vi "Process Data XYGraph.vi"(5 "Queue":refnum<queue>) -> ()   [LabVIEW 2013, in "main.lvlib"]
uses:
  main.lvlib
  Controls/Enum Variables.ctl
  Controls/Enum User Events.ctl
  Controls/Enum Process Data.ctl
  CreatePDF XYGraph.vi
panel:
  out "Blue":cluster{"Pressure":dbl[], "Graph":dbl[]}(graph)
  out "Blue index":dbl format="%d%%"
  in  "ResetBlueBtn":bool
  in  "ZoomBlueBtn":bool
  out "Blue Pressure":dbl
  out "Red":cluster{"Pressure":dbl[], "Graph":dbl[]}(graph)
  out "Armpressure":dbl
  in  "System Stop Button":bool
  in  "GraphSelection(Red:F)":bool
  in  "Cursor Mode":bool
  in  "ResetFrontImage":bool
  out "Red index":dbl format="%d%%"
  out "Red Pressure":dbl
  in  "ResetRedBtn":bool
  in  "ZoomRedBtn":bool
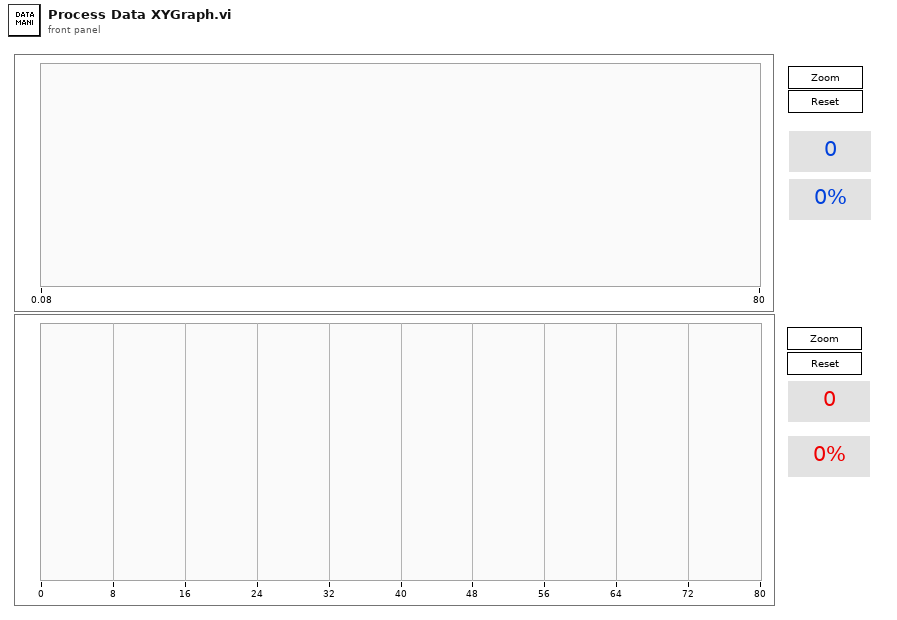
[diagram p1: front panel]
types:
  T1 = typedef "main.lvlib/Enum Process Data.ctl" = enum16{"Init", "Set Cursor Mode", "Set Data Path", "Get All"}
  T2 = typedef "main.lvlib/Enum Variables.ctl" = enum16{"SetAcqFilter", "GetAcqFilter", "Set Filter", "Get Filter", "Set Height", "Get Height", "Set Blue Pressure", "Get Blue Pressure", "Set Red Pressure", "Get Red Pressure", "Init", "Reset Pressure", "Set Red Cursors", "Get Red Cursors", "Set Blue Cursors", "Get Blue Cursors", "Set Language", "Get Language", "Set Active Graphs", "Get ActiveGraphs", "Set Method", "Get Method", "Set Encryption", "Get Encryption", "Set ExcelVersion", "Get ExcelVersion", "Set DICOM Avail", "Get DICOM Avail", "Set DICOM Encode", "Get DICOM Encode", "Set JournalExport", "Get JournalExport", "Set Sequence", "Get Sequence", "Set DAQ Connected", "Get DAQ Connected", "Set Current Graph", "Get Current Graph", "Set General Settings", "Get Hyphenation", "Set Arm Calc Method", "Get Arm Calc Method", "Set Dicom Tags", "Get Dicom Tags", "Set BT Serial", "Get BT Serial", "Set BT Accepted Serials", "Get BT Accepted Serials", "Get BT License", "Set BT License"}
  T3 = typedef "main.lvlib/Enum User Events.ctl" = enum16{"User Event", "Init"}
  T4 = typedef "LVPoint32TypeDef.ctl" = cluster{"Horizontal":i32, "Vertical":i32}
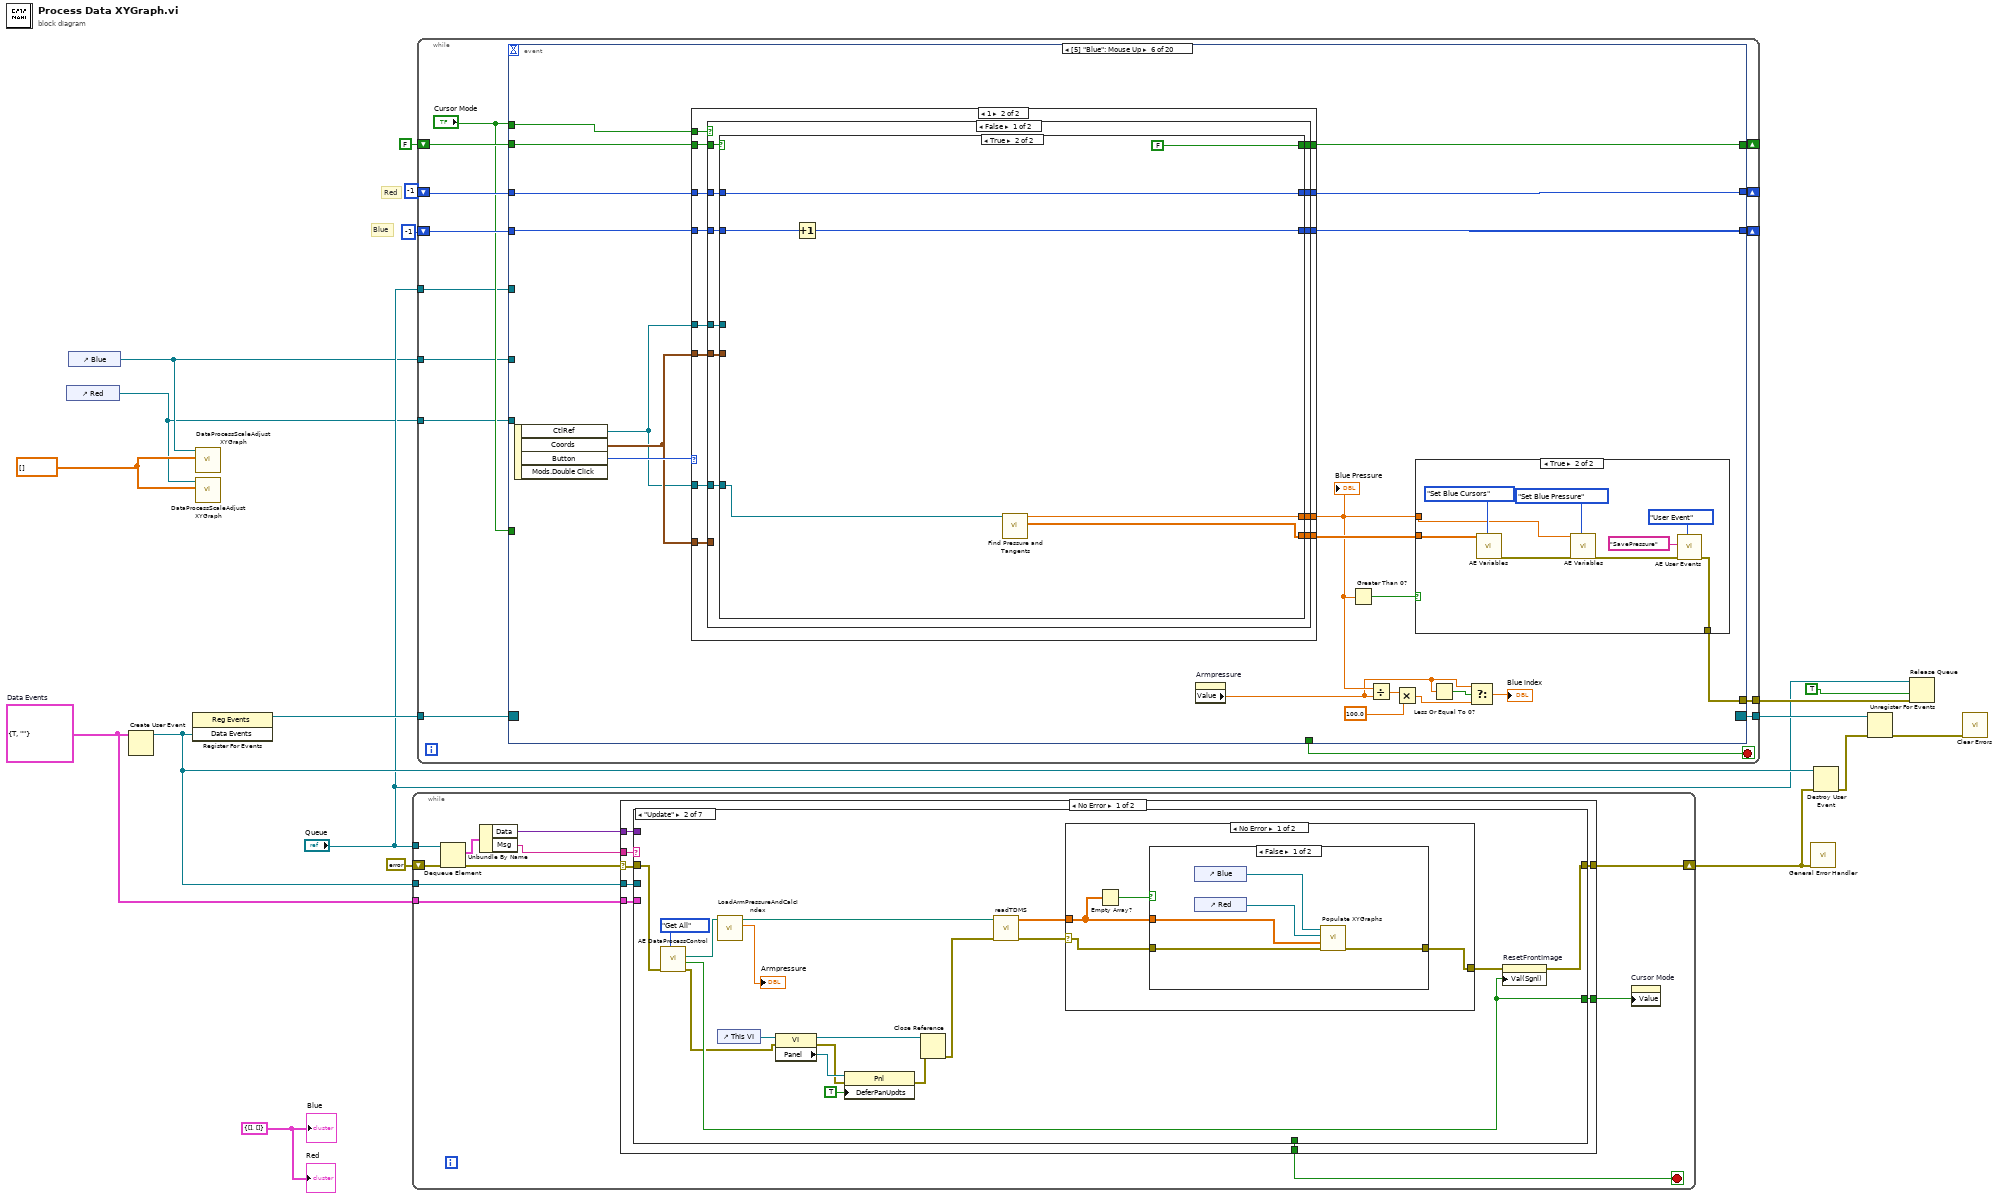
[diagram p0: block diagram]
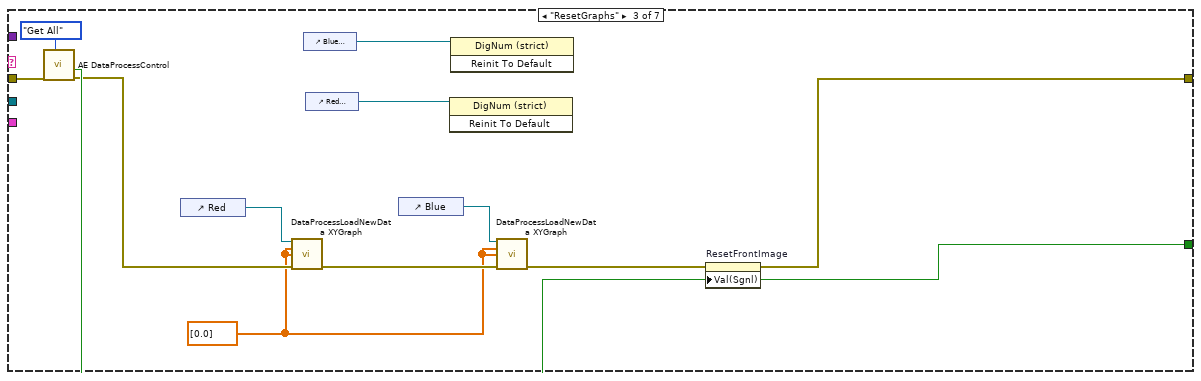
[diagram p5: hidden frame]
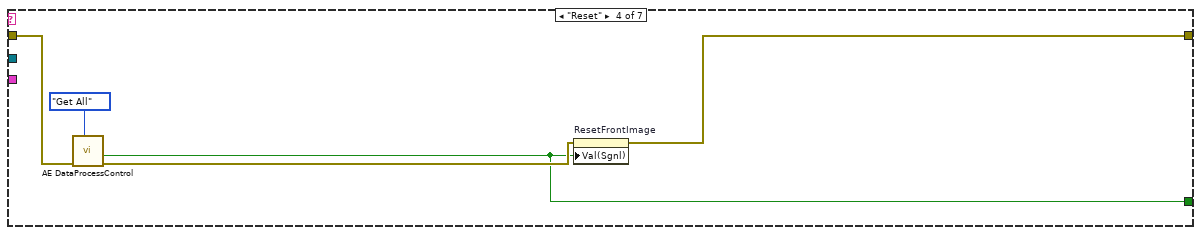
[diagram p6: hidden frame]
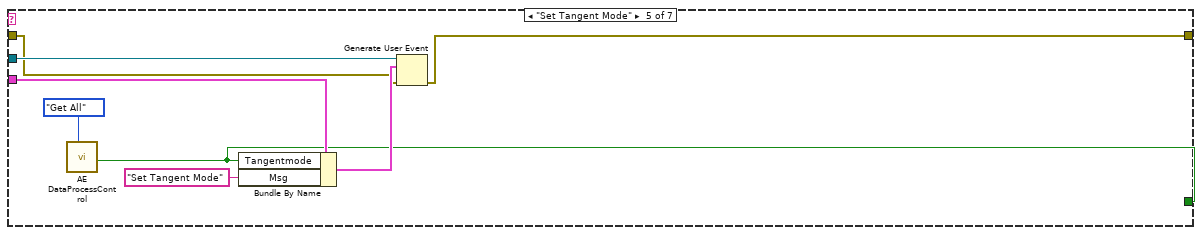
[diagram p7: hidden frame]
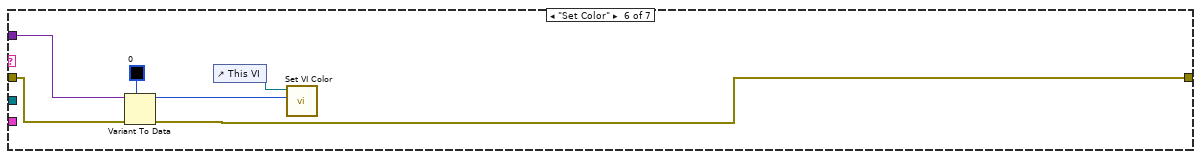
[diagram p8: hidden frame]
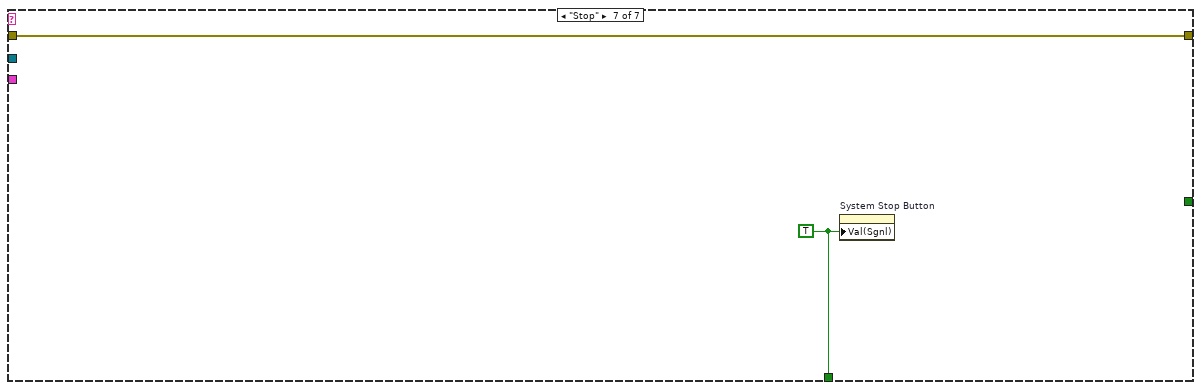
[diagram p9: hidden frame]
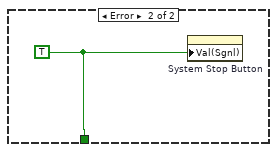
[diagram p10: hidden frame]
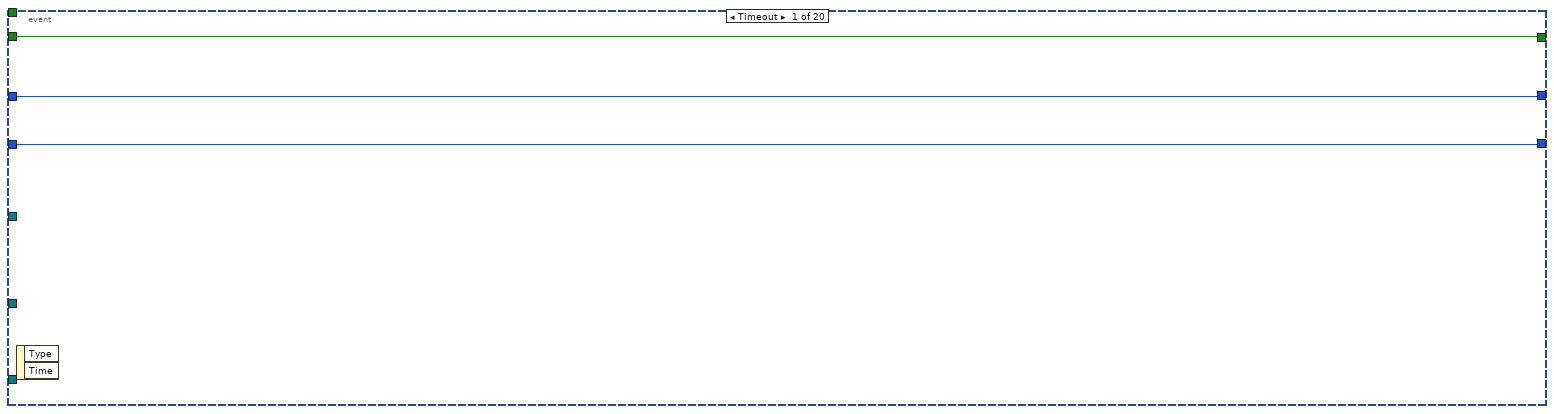
[diagram p11: hidden frame]
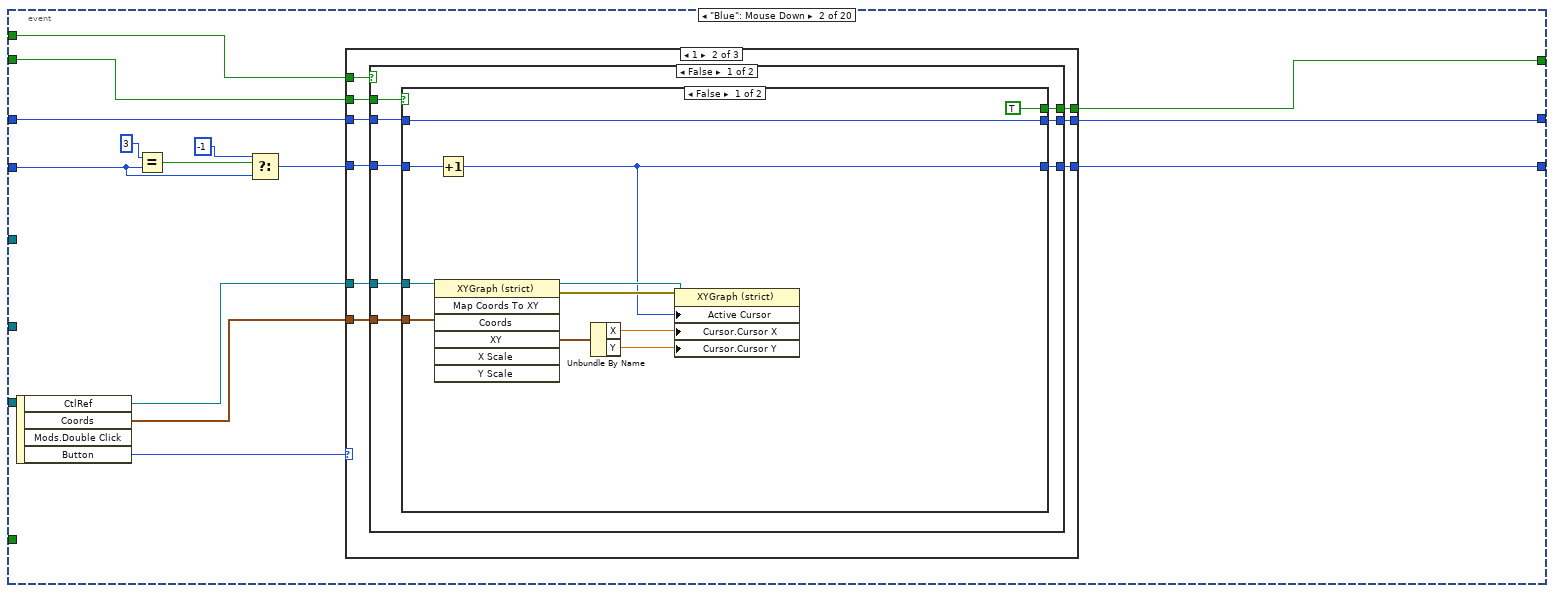
[diagram p12: hidden frame]
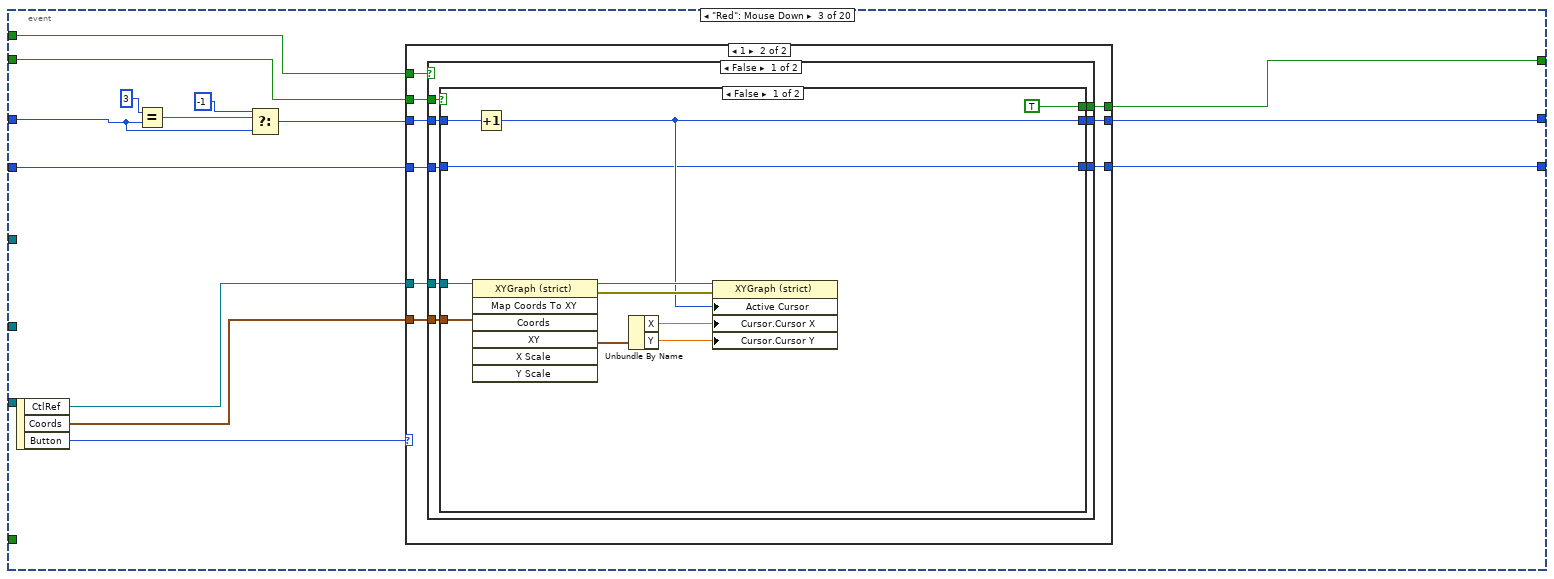
[diagram p17: hidden frame]
diagram:
  w1 = cluster{"Pressure":dbl[], "Graph":dbl[]} {"Pressure"=[], "Graph"=[]}
  w5 = dbl[] []
  w12 = cluster{"Tangentmode":bool, "Msg":string} {"Tangentmode"=TRUE, "Msg"=""}  # Data Events
  # "Blue"
  # "Red"
  n1 = control-ref of="Red"() -> (w3:refnum<vi>)
  n2 = control-ref of="Blue"() -> (w4:refnum<vi>)
  n3 = Create User Event(user event datatype=w12) -> (user event=w8:refnum<user-event>)  [unwired: 1 in, 1 out]
  n4 = register-events(w8) -> (reference out=w13:refnum<event-registration>)  [unwired: 2 in, 1 out]
  n5 = call "DataProcessScaleAdjust XYGraph.vi"(10:"Graph"=w5, 11:"Graph"=w4) -> ()  [unwired: 8 in, 2 out]
  n6 = call "DataProcessScaleAdjust XYGraph.vi"(10:"Graph"=w5, 11:"Graph"=w3) -> ()  [unwired: 8 in, 2 out]
  n7 = while {
    tunnel: "Queue" -> [w29]
    shift-right: [w28] -> w9
    shift-left: errorcluster {"status"=FALSE, "code"=0, "source"=""} ("error IO") -> [w27]
    tunnel: w8 -> [w25]
    tunnel: w12 -> [w24]
    stop <- w20 stop-if-true
    n8 = Dequeue Element(queue=w29, error in (no error)=w27) -> (element=w23:cluster{"Msg":string, "Data":variant}, error out=w19:errorcluster)  [unwired: 1 in, 2 out]
    n9 = Unbundle By Name(w23) -> ("Data"=w21:variant, "Msg"=w22:string)
    n10 = case shown="No Error" w19 {
      selector: w19 -> [w30 _]
      tunnel: [w37 _] -> w28
      tunnel: [w36 _] -> w26
      tunnel: w25 -> [w35 _]
      tunnel: w24 -> [w34 _]
      tunnel: w22 -> [w33 _]
      tunnel: w21 -> [w32 _]
      tunnel: [w31 w101] -> w20
      frame No Error {
        n11 = case shown="\"Update\"" w33 {
          tunnel: w30 -> [w38 w51 w73 w82 w86 w94 w100]
          tunnel: [w38 w39 w75 w84 w85 w93 w100] -> w37
          tunnel: [_ w48 w72 w80 w87 _ _] -> w36
          tunnel: [_ _ _ _ _ _ w99] -> w31
          tunnel: w35 -> [_ _ _ _ w92 _ _]
          tunnel: w34 -> [_ _ _ _ w90 _ _]
          tunnel: w32 -> [_ _ _ _ _ w97 _]
          frame "", Default {
          }
          frame "Update" {
            n12 = call "AE DataProcessControl.vi"("Action"=Enum_Process_Data."Get All", "error in (no error)"=w51) -> ("error out"=w41:errorcluster, "Cursor Mode Out"=w48:bool, "Data Path Out"=w50:path)  [unwired: 7 in]
            n13 = call "LoadArmPressureAndCalcIndex.vi"("Path"=w50) -> ("Armpressure"=→"Armpressure":dbl, "Path Out"=w52:path)  [unwired: 8 in, 1 out]
            n14 = control-ref of="This VI"() -> (w46:refnum<vi>)
            n15 = property class="VI"(reference=w46, error in=w41) -> (reference out=w47:refnum<vi>, error out=w43:errorcluster, "Panel"=w45:refnum<vi>)
            n16 = property class="Pnl"(reference=w45, error in=w43, "DeferPanUpdts"=TRUE ("Defer Panel Updates")) -> (error out=w44:errorcluster)  [unwired: 1 out]
            n17 = Close Reference(reference=w47, error in (no error)=w44) -> (error out=w40:errorcluster)
            n18 = call "readTDMS.vi"("error in (no error)"=w40, "Path Out"=w52) -> ("error out"=w55:errorcluster, "Array"=w56:dbl[][])  [unwired: 8 in]
            n19 = case shown="No Error" w55 {
              selector: w55 -> [w59 w67]
              tunnel: w56 -> [w58 _]
              tunnel: [w60 w67] -> w54
              frame No Error {
                n20 = Empty Array?(array=w58) -> (empty?=w57:bool)
                n21 = case shown="False" w57 {
                  tunnel: [w65 w66] -> w60
                  tunnel: w58 -> [w63 _]
                  tunnel: w59 -> [w61 w66]
                  frame False {
                    n22 = control-ref of="Blue"() -> (w64:refnum<vi>)
                    n23 = control-ref of="Red"() -> (w62:refnum<vi>)
                    n24 = call "Populate XYGraphs.vi"("error in (no error)"=w61, "Array"=w63, "Red"=w62, "Blue"=w64) -> ("error out"=w65:errorcluster)  [unwired: 7 in]
                  }
                  frame True {
                  }
                }
              }
              frame Error {
              }
            }
            n25 = property on="ResetFrontImage" class="Bool (strict)"(error in=w54, "Val(Sgnl)"=w48) -> (error out=w39:errorcluster)  [unwired: 1 in, 1 out]
          }
          frame "ResetGraphs" {
            w68 = dbl[] [0.0]
            n26 = call "AE DataProcessControl.vi"("Action"=Enum_Process_Data."Get All", "error in (no error)"=w73) -> ("error out"=w70:errorcluster, "Cursor Mode Out"=w72:bool)  [unwired: 7 in, 1 out]
            n27 = control-ref of="Red"() -> (w69:refnum<vi>)
            n28 = call "DataProcessLoadNewData XYGraph.vi"(0:"Graph"=w69, 5:"Graph"=w68, "Pressure"=w68, "error in (no error)"=w70) -> ("error out"=w71:errorcluster)  [unwired: 10 in, 1 out]
            n29 = control-ref of="Blue Pressure"() -> (w77:refnum<vi>)
            n30 = control-ref of="Red Pressure"() -> (w76:refnum<vi>)
            n31 = control-ref of="Blue"() -> (w78:refnum<vi>)
            n32 = invoke class="DigNum (strict)" method="Reinit To Default"(reference=w76) -> ()  [unwired: 2 in, 3 out]
            n33 = invoke class="DigNum (strict)" method="Reinit To Default"(reference=w77) -> ()  [unwired: 2 in, 3 out]
            n34 = call "DataProcessLoadNewData XYGraph.vi"(0:"Graph"=w78, 5:"Graph"=w68, "Pressure"=w68, "error in (no error)"=w71) -> ("error out"=w79:errorcluster)  [unwired: 10 in, 1 out]
            n35 = property on="ResetFrontImage" class="Bool (strict)"(error in=w79, "Val(Sgnl)"=w72) -> (error out=w75:errorcluster)  [unwired: 1 in, 1 out]
          }
          frame "Reset" {
            n36 = call "AE DataProcessControl.vi"("Action"=Enum_Process_Data."Get All", "error in (no error)"=w82) -> ("error out"=w81:errorcluster, "Cursor Mode Out"=w80:bool)  [unwired: 7 in, 1 out]
            n37 = property on="ResetFrontImage" class="Bool (strict)"(error in=w81, "Val(Sgnl)"=w80) -> (error out=w84:errorcluster)  [unwired: 1 in, 1 out]
          }
          frame "Set Tangent Mode" {
            n38 = call "AE DataProcessControl.vi"("Action"=Enum_Process_Data."Get All") -> ("Cursor Mode Out"=w87:bool)  [unwired: 8 in, 2 out]
            n39 = Bundle By Name(cluster=w90, "Tangentmode"=w87, "Msg"="Set Tangent Mode") -> (w89:cluster{"Tangentmode":bool, "Msg":string})
            n40 = Generate User Event(user event=w92, event data cluster=w89, error in=w86) -> (error out=w85:errorcluster)  [unwired: 1 in, 1 out]
          }
          frame "Set Color" {
            n41 = Variant To Data(error in=w94, type=u32 0, Variant=w97) -> (data=w96:u32, error out=w93:errorcluster)
            n42 = control-ref of="This VI"() -> (w98:refnum<vi>)
            n43 = call "Set VI Color.vi"("Pane Color"=w96, "VI in"=w98) -> ()  [unwired: 10 in]
          }
          frame "Stop" {
            w99 = TRUE
            n44 = property on="System Stop Button" class="Bool (strict)"("Val(Sgnl)"=w99) -> ()  [unwired: 2 in, 2 out]
          }
        }
      }
      frame Error {
        w101 = TRUE
        n45 = property on="System Stop Button" class="Bool (strict)"("Val(Sgnl)"=w101) -> ()  [unwired: 2 in, 2 out]
      }
    }
    n46 = property on="Cursor Mode" class="Bool (strict)"("Value"=w26) -> ()  [unwired: 2 in, 2 out]
  }
  n47 = while {
    shift-right: [w114] -> _
    shift-left: -1 -> [w111]
    shift-right: [w113] -> _
    shift-left: -1 -> [w112]
    shift-right: [w110] -> _
    shift-left: FALSE -> [w109]
    tunnel: w4 -> [w107]
    tunnel: w3 -> [w106]
    tunnel: "Queue" -> [w105]
    tunnel: [w104] -> w14
    tunnel: w13 -> [w103]
    tunnel: [w102] -> w11
    stop <- w115 stop-if-true
    n48 = event shown="[5] \"Blue\": Mouse Up" {
      selector: w103 -> [_ _ _ _ _ _ _ _ _ _ _ _ _ _ _ _ _ _ _ _]
      dyn-events: [_ _ _ _ _ _ _ _ _ _ _ _ _ _ _ _ _ _ _ _] -> w102
      timeout: _ -> [_ _ _ _ _ _ _ _ _ _ _ _ _ _ _ _ _ _ _ _]
      tunnel: [_ _ _ _ _ _ _ _ _ _ _ _ _ "System Stop Button" _ _ _ _ _ _] -> w115
      tunnel: [w118 w130 w184 w235 w262 w297 w369 w424 w447 w472 w499 w523 w551 w555 w560 w577 w596 w619 w637 w651] -> w114
      tunnel: [w117 w129 w183 w234 w261 w295 w367 w427 w450 w471 w498 w522 w550 w554 w561 w576 w595 w618 w638 w650] -> w113
      tunnel: w112 -> [w117 w124 w177 w227 w254 w292 w364 w428 w451 w471 w498 w522 w550 w554 w561 w576 w595 w618 w638 w650]
      tunnel: w111 -> [w118 w128 w178 w233 w256 w296 w368 w425 w448 w472 w499 w523 w551 w555 w560 w577 w596 w619 w637 w651]
      tunnel: [w116 w121 w174 w232 w260 w293 w365 w426 w449 w470 w500 w521 w552 w553 w559 w578 w597 w620 w639 w652] -> w110
      tunnel: w109 -> [w116 w122 w176 w232 w260 w294 w366 w429 w452 w470 w500 w521 w552 w553 w559 w578 w597 w620 w639 w652]
      tunnel: "Cursor Mode" -> [_ w120 w175 _ _ w291 w363 w423 w446 _ _ _ _ _ _ _ _ _ _ _]
      tunnel: "Cursor Mode" -> [_ _ _ w224 w251 _ _ _ _ _ _ _ _ _ _ _ _ _ _ _]
      tunnel: w107 -> [_ _ _ _ _ _ _ _ _ _ w474 w527 _ _ _ w574 _ _ _ _]
      tunnel: w106 -> [_ _ _ _ _ _ _ _ _ _ w473 w526 _ _ w557 _ _ _ _ _]
      tunnel: w105 -> [_ _ _ _ _ _ _ _ _ _ _ _ _ _ w558 w575 _ _ _ w654]
      tunnel: [_ _ _ _ _ w278 _ _ _ _ _ _ _ _ _ _ _ _ _ _] -> w104
      event Timeout {
        n49 = event-data() -> ()  [unwired: 1 in, 2 out]
      }
      event "Blue": Mouse Down {
        n50 = event-data() -> ("CtlRef"=w132:refnum<vi>, "Coords"=w131:T4, "Button"=w119:u16)  [unwired: 1 in, 1 out]
        n51 = Equal?(x=3, y=w124) -> (x = y?=w125:bool)
        n52 = Select(t=-1, s=w125, f=w124) -> (s? t:f=w123:i32)
        n53 = case shown="1" w119 {
          tunnel: w132 -> [_ w144 _]
          tunnel: w131 -> [_ w143 _]
          tunnel: [w135 w142 w171] -> w130
          tunnel: [w134 w141 w170] -> w129
          tunnel: w128 -> [w135 w140 w171]
          tunnel: w123 -> [w134 w139 w170]
          tunnel: w122 -> [w133 w138 w172]
          tunnel: [w133 w137 w172] -> w121
          tunnel: w120 -> [_ w136 _]
          frame 0, Default {
          }
          frame 1 {
            n54 = case shown="False" w136 {
              tunnel: w144 -> [w152 _]
              tunnel: w143 -> [w151 _]
              tunnel: [w150 w169] -> w142
              tunnel: [w149 w168] -> w141
              tunnel: w140 -> [w148 w169]
              tunnel: w139 -> [w147 w168]
              tunnel: w138 -> [w146 w167]
              tunnel: [w145 w167] -> w137
              frame False {
                n55 = case shown="False" w146 {
                  selector: w146 -> [_ w164]
                  tunnel: w152 -> [w163 _]
                  tunnel: w151 -> [w162 _]
                  tunnel: w147 -> [w155 w166]
                  tunnel: [w154 w166] -> w149
                  tunnel: w148 -> [w156 w165]
                  tunnel: [w156 w165] -> w150
                  tunnel: [TRUE w164] -> w145
                  frame False {
                    n56 = invoke class="XYGraph (strict)" method="Map Coords To XY"(reference=w163, "Coords"=w162) -> (reference out=w161:refnum<vi>, error out=w160:errorcluster, "XY"=w159:cluster{"X":dbl, "Y":dbl})  [unwired: 5 in, 4 out]
                    n57 = Increment(x=w155) -> (x+1=w154:i32)
                    n58 = Unbundle By Name(w159) -> ("X"=w158:dbl, "Y"=w157:dbl)
                    n59 = property class="XYGraph (strict)"(reference=w161, error in=w160, "Active Cursor"=w154, "Cursor.Cursor X"=w158, "Cursor.Cursor Y"=w157) -> ()  [unwired: 2 out]
                  }
                  frame True {
                  }
                }
              }
              frame True {
              }
            }
          }
          frame 2 {
          }
        }
      }
      event "Red": Mouse Down {
        n60 = event-data() -> ("CtlRef"=w186:refnum<vi>, "Coords"=w185:T4, "Button"=w173:u16)  [unwired: 1 in]
        n61 = Equal?(x=3, y=w178) -> (x = y?=w180:bool)
        n62 = Select(t=-1, s=w180, f=w178) -> (s? t:f=w179:i32)
        n63 = case shown="1" w173 {
          tunnel: w186 -> [_ w198]
          tunnel: w185 -> [_ w197]
          tunnel: [w188 w196] -> w184
          tunnel: [w187 w195] -> w183
          tunnel: w179 -> [w188 w194]
          tunnel: w177 -> [w187 w193]
          tunnel: w176 -> [w189 w192]
          tunnel: w175 -> [_ w191]
          tunnel: [w189 w190] -> w174
          frame 0, Default {
          }
          frame 1 {
            n64 = case shown="False" w191 {
              tunnel: w198 -> [w206 _]
              tunnel: w197 -> [w205 _]
              tunnel: [w204 w223] -> w196
              tunnel: [w203 w221] -> w195
              tunnel: w194 -> [w202 w223]
              tunnel: w193 -> [w201 w221]
              tunnel: w192 -> [w200 w222]
              tunnel: [w199 w222] -> w190
              frame False {
                n65 = case shown="False" w200 {
                  selector: w200 -> [_ w218]
                  tunnel: w206 -> [w217 _]
                  tunnel: w205 -> [w216 _]
                  tunnel: w201 -> [w208 w220]
                  tunnel: [w208 w220] -> w203
                  tunnel: w202 -> [w210 w219]
                  tunnel: [w209 w219] -> w204
                  tunnel: [TRUE w218] -> w199
                  frame False {
                    n66 = invoke class="XYGraph (strict)" method="Map Coords To XY"(reference=w217, "Coords"=w216) -> (reference out=w215:refnum<vi>, error out=w214:errorcluster, "XY"=w213:cluster{"X":dbl, "Y":dbl})  [unwired: 5 in, 4 out]
                    n67 = Increment(x=w210) -> (x+1=w209:i32)
                    n68 = Unbundle By Name(w213) -> ("X"=w212:dbl, "Y"=w211:dbl)
                    n69 = property class="XYGraph (strict)"(reference=w215, error in=w214, "Active Cursor"=w209, "Cursor.Cursor X"=w212, "Cursor.Cursor Y"=w211) -> ()  [unwired: 2 out]
                  }
                  frame True {
                  }
                }
              }
              frame True {
              }
            }
          }
        }
      }
      event "Blue": Mouse Move {
        # "Drawing the line between the first point and the mouse"
        n70 = event-data() -> ("CtlRef"=w226:refnum<vi>, "Coords"=w225:T4)  [unwired: 1 in]
        n71 = Equal?(x=3, y=w227) -> (x = y?=w229:bool)
        n72 = Select(t=-1, s=w229, f=w227) -> (s? t:f=w228:i32)
        n73 = case shown="True" w232 {
          tunnel: w226 -> [_ w250]
          tunnel: w225 -> [_ w249]
          tunnel: w228 -> [w239 w241]
          tunnel: [w239 w241] -> w234
          tunnel: w233 -> [w238 w243]
          tunnel: [w238 w243] -> w235
          frame False {
          }
          frame True {
            n74 = invoke class="XYGraph (strict)" method="Map Coords To XY"(reference=w250, "Coords"=w249) -> (reference out=w248:refnum<vi>, error out=w247:errorcluster, "XY"=w246:cluster{"X":dbl, "Y":dbl})  [unwired: 5 in, 4 out]
            n75 = Unbundle By Name(w246) -> ("X"=w245:dbl, "Y"=w244:dbl)
            n76 = Increment(x=w241) -> (x+1=w242:i32)
            n77 = property class="XYGraph (strict)"(reference=w248, error in=w247, "Active Cursor"=w242, "Cursor.Cursor X"=w245, "Cursor.Cursor Y"=w244) -> (reference out=w240:refnum<vi>)  [unwired: 1 out]
            n78 = call "DrawCursorLines XYGraph.vi"("CtlRef"=w240) -> ()  [unwired: 9 in, 2 out]
          }
        }
        n79 = case shown="True" w224 {
          tunnel: w226 -> [_ w236]
          tunnel: w225 -> [_ w237]
          frame False {
          }
          frame True {
            n80 = call "UpdateMovingCursor XYGraph.vi"("Coords"=w237, "CtlRef"=w236) -> ()  [unwired: 8 in]
          }
        }
      }
      event "Red": Mouse Move {
        n81 = event-data() -> ("CtlRef"=w253:refnum<vi>, "Coords"=w252:T4)  [unwired: 1 in]
        n82 = Equal?(x=3, y=w256) -> (x = y?=w257:bool)
        n83 = Select(t=-1, s=w257, f=w256) -> (s? t:f=w255:i32)
        n84 = case shown="True" w260 {
          tunnel: w253 -> [_ w277]
          tunnel: w252 -> [_ w276]
          tunnel: w254 -> [w266 w269]
          tunnel: [w266 w269] -> w261
          tunnel: w255 -> [w265 w268]
          tunnel: [w265 w268] -> w262
          frame False {
          }
          frame True {
            n85 = invoke class="XYGraph (strict)" method="Map Coords To XY"(reference=w277, "Coords"=w276) -> (reference out=w275:refnum<vi>, error out=w274:errorcluster, "XY"=w273:cluster{"X":dbl, "Y":dbl})  [unwired: 5 in, 4 out]
            n86 = Unbundle By Name(w273) -> ("X"=w272:dbl, "Y"=w271:dbl)
            n87 = Increment(x=w268) -> (x+1=w270:i32)
            n88 = property class="XYGraph (strict)"(reference=w275, error in=w274, "Active Cursor"=w270, "Cursor.Cursor X"=w272, "Cursor.Cursor Y"=w271) -> (reference out=w267:refnum<vi>)  [unwired: 1 out]
            n89 = call "DrawCursorLines XYGraph.vi"("CtlRef"=w267) -> ()  [unwired: 9 in, 2 out]
          }
        }
        n90 = case shown="True" w251 {
          tunnel: w253 -> [w264 _]
          tunnel: w252 -> [w263 _]
          frame True {
            n91 = call "UpdateMovingCursor XYGraph.vi"("Coords"=w263, "CtlRef"=w264) -> ()  [unwired: 8 in]
          }
          frame False {
          }
        }
      }
      event "Blue": Mouse Up {
        n92 = event-data() -> ("CtlRef"=w288:refnum<vi>, "Coords"=w289:T4, "Button"=w290:u16)  [unwired: 1 in, 1 out]
        n93 = case shown="1" w290 {
          tunnel: [w300 w313] -> w297
          tunnel: w296 -> [w300 w312]
          tunnel: [w299 w311] -> w295
          tunnel: w294 -> [w298 w310]
          tunnel: [w298 w309] -> w293
          tunnel: w292 -> [w299 w308]
          tunnel: w291 -> [_ w307]
          tunnel: w288 -> [_ w306]
          tunnel: w289 -> [_ w305]
          tunnel: [_ w304] -> w283
          tunnel: w289 -> [_ w303]
          tunnel: w288 -> [_ w302]
          tunnel: [_ w301] -> w286
          frame 0, Default {
          }
          frame 1 {
            n94 = case shown="False" w307 {
              tunnel: w305 -> [w324 _]
              tunnel: [w323 w340] -> w313
              tunnel: w312 -> [w322 w340]
              tunnel: [w321 w339] -> w311
              tunnel: w306 -> [w320 _]
              tunnel: w310 -> [w319 w341]
              tunnel: [w318 w341] -> w309
              tunnel: w308 -> [w317 w339]
              tunnel: w302 -> [w316 w338]
              tunnel: [w315 w336] -> w304
              tunnel: w303 -> [_ w337]
              tunnel: [w314 _] -> w301
              frame False {
                n95 = case shown="True" w319 {
                  selector: w319 -> [w326 _]
                  tunnel: w320 -> [_ _]
                  tunnel: w324 -> [_ _]
                  tunnel: w317 -> [w328 w334]
                  tunnel: [w328 w333] -> w321
                  tunnel: w322 -> [w327 w335]
                  tunnel: [w327 w335] -> w323
                  tunnel: [w326 FALSE] -> w318
                  tunnel: w316 -> [_ w331]
                  tunnel: [0.0 w329] -> w315
                  tunnel: [_ w330] -> w314
                  frame False {
                  }
                  frame True {
                    n96 = Increment(x=w334) -> (x+1=w333:i32)
                    n97 = call "Find Pressure and Tangents.vi"("XYGraph in"=w331) -> ("Tangents"=w330:dbl[][], "Pressure"=w329:dbl)  [unwired: 9 in]
                  }
                }
              }
              frame True {
                n98 = call "GetPressureAtMouse XYGraph.vi"("Coords"=w337, "GraphRefnum"=w338) -> ("Numeric"=w336:dbl)  [unwired: 1 out]
              }
            }
          }
        }
        "Blue Pressure" <- w283
        n99 = property on="Armpressure" class="DigNum (strict)"() -> ("Value"=w279:dbl)  [unwired: 2 in, 2 out]
        n100 = Greater Than 0?(x=w283) -> (x > 0?=w287:bool)
        n101 = Divide(x=w283, y=w279) -> (x/y=w285:dbl)
        n102 = Multiply(x=w285, y=100.0) -> (x*y=w281:dbl)
        n103 = case shown="True" w287 {
          tunnel: w283 -> [_ w344]
          tunnel: w286 -> [_ w345]
          tunnel: [_ w343] -> w278
          frame False {
          }
          frame True {
            n104 = call "AE Variables.vi"("VariantIn"=w345, "Action"=Enum_Variables."Set Blue Cursors") -> ("error out"=w347:errorcluster)  [unwired: 10 in, 7 out]
            n105 = call "AE Variables.vi"("VariantIn"=w344, "error in (no error)"=w347, "Action"=Enum_Variables."Set Blue Pressure") -> ("error out"=w342:errorcluster)  [unwired: 9 in, 7 out]
            n106 = call "AE User Events.vi"("Action"=Enum_User_Events."User Event", "error in (no error)"=w342, "User Event"="SavePressure") -> ("error out"=w343:errorcluster)  [unwired: 7 in, 1 out]
          }
        }
        n107 = Less Or Equal To 0?(x=w279) -> (x <= 0?=w280:bool)
        n108 = Select(t=w279, s=w280, f=w281) -> (s? t:f=→"Blue index":dbl)
      }
      event "Red": Mouse Up {
        n109 = event-data() -> ("CtlRef"=w359:refnum<vi>, "Coords"=w360:T4, "Button"=w361:u16)  [unwired: 1 in, 1 out]
        n110 = case shown="1" w361 {
          tunnel: [w372 w385] -> w369
          tunnel: w368 -> [w372 w384]
          tunnel: [w371 w383] -> w367
          tunnel: w366 -> [w370 w382]
          tunnel: [w370 w381] -> w365
          tunnel: w364 -> [w371 w380]
          tunnel: w363 -> [_ w379]
          tunnel: w359 -> [_ w378]
          tunnel: w360 -> [_ w377]
          tunnel: [_ w376] -> w357
          tunnel: w360 -> [_ w375]
          tunnel: w359 -> [_ w374]
          tunnel: [_ w373] -> w358
          frame 0, Default {
          }
          frame 1 {
            n111 = case shown="False" w379 {
              tunnel: w377 -> [w396 _]
              tunnel: [w387 w412] -> w385
              tunnel: w384 -> [w395 w412]
              tunnel: [w394 w411] -> w383
              tunnel: w378 -> [w393 _]
              tunnel: w382 -> [w392 w413]
              tunnel: [w391 w413] -> w381
              tunnel: w380 -> [w390 w411]
              tunnel: w374 -> [w389 w410]
              tunnel: [w388 w408] -> w376
              tunnel: w375 -> [_ w409]
              tunnel: [w386 _] -> w373
              frame False {
                n112 = case shown="True" w392 {
                  selector: w392 -> [w398 _]
                  tunnel: w393 -> [_ _]
                  tunnel: w396 -> [_ _]
                  tunnel: w390 -> [w400 w406]
                  tunnel: [w400 w406] -> w394
                  tunnel: w395 -> [w399 w405]
                  tunnel: [w399 w404] -> w387
                  tunnel: [w398 FALSE] -> w391
                  tunnel: w389 -> [_ w403]
                  tunnel: [0.0 w402] -> w388
                  tunnel: [_ w401] -> w386
                  frame False {
                  }
                  frame True {
                    n113 = Increment(x=w405) -> (x+1=w404:i32)
                    n114 = call "Find Pressure and Tangents.vi"("XYGraph in"=w403) -> ("Tangents"=w401:dbl[][], "Pressure"=w402:dbl)  [unwired: 9 in]
                  }
                }
              }
              frame True {
                n115 = call "GetPressureAtMouse XYGraph.vi"("Coords"=w409, "GraphRefnum"=w410) -> ("Numeric"=w408:dbl)  [unwired: 1 out]
              }
            }
          }
        }
        "Red Pressure" <- w357
        n116 = property on="Armpressure" class="DigNum (strict)"() -> ("Value"=w351:dbl)  [unwired: 2 in, 2 out]
        n117 = Greater Than 0?(x=w357) -> (x > 0?=w362:bool)
        n118 = Divide(x=w357, y=w351) -> (x/y=w356:dbl)
        n119 = Multiply(x=w356, y=100.0) -> (x*y=w352:dbl)
        n120 = case shown="True" w362 {
          tunnel: w357 -> [_ w418]
          tunnel: w358 -> [_ w415]
          frame False {
          }
          frame True {
            n121 = call "AE Variables.vi"("VariantIn"=w415, "Action"=Enum_Variables."Set Red Cursors") -> ("error out"=w417:errorcluster)  [unwired: 10 in, 7 out]
            n122 = To Variant(anything=w418) -> (Variant=w419:variant)
            n123 = call "AE Variables.vi"("VariantIn"=w419, "error in (no error)"=w417, "Action"=Enum_Variables."Set Red Pressure") -> ("error out"=w414:errorcluster)  [unwired: 9 in, 7 out]
            n124 = call "AE User Events.vi"("Action"=Enum_User_Events."User Event", "error in (no error)"=w414, "User Event"="SavePressure") -> ()  [unwired: 7 in, 2 out]
          }
        }
        n125 = Less Or Equal To 0?(x=w351) -> (x <= 0?=w354:bool)
        n126 = Select(t=w351, s=w354, f=w352) -> (s? t:f=→"Red index":dbl)
      }
      event "Blue": Mouse Leave {
        n127 = event-data() -> ()  [unwired: 1 in, 1 out]
        n128 = case shown="False" w423 {
          tunnel: w429 -> [w435 w445]
          tunnel: w428 -> [w434 w443]
          tunnel: [w433 w443] -> w427
          tunnel: [w432 w445] -> w426
          tunnel: w425 -> [w431 w444]
          tunnel: [w430 w444] -> w424
          frame False {
            n129 = case shown="False" w435 {
              selector: w435 -> [w437 _]
              tunnel: w434 -> [w438 w442]
              tunnel: [w438 w441] -> w433
              tunnel: [w437 FALSE] -> w432
              tunnel: w431 -> [w436 w439]
              tunnel: [w436 w439] -> w430
              frame False {
              }
              frame True {
                n130 = Increment(x=w442) -> (x+1=w441:i32)
              }
            }
          }
          frame True {
          }
        }
      }
      event "Red": Mouse Leave {
        n131 = event-data() -> ()  [unwired: 1 in, 1 out]
        n132 = case shown="False" w446 {
          tunnel: w452 -> [w458 w468]
          tunnel: w451 -> [w457 w466]
          tunnel: [w456 w466] -> w450
          tunnel: [w455 w468] -> w449
          tunnel: w448 -> [w454 w467]
          tunnel: [w453 w467] -> w447
          frame False {
            n133 = case shown="False" w458 {
              selector: w458 -> [w460 _]
              tunnel: w457 -> [w461 w464]
              tunnel: [w461 w464] -> w456
              tunnel: [w460 FALSE] -> w455
              tunnel: w454 -> [w459 w463]
              tunnel: [w459 w462] -> w453
              frame False {
              }
              frame True {
                n134 = Increment(x=w463) -> (x+1=w462:i32)
              }
            }
          }
          frame True {
          }
        }
      }
      event "Blue": event type 3.0.x80000027 {
        n135 = event-data() -> ()  [unwired: 1 in, 8 out]
        n136 = event-data("Discard?"=TRUE) -> ()  [unwired: 1 in, 1 out]
      }
      event "ResetFrontImage": Value Change {
        n137 = event-data() -> ()  [unwired: 1 in, 1 out]
        n138 = Build Array(w474, w473) -> (w494:refnum<vi>[])
        n139 = for {
          tunnel: picture data[5B] ("Plot Images:Front") -> [w508]
          tunnel: w494 -> [w507] mode=indexing
          tunnel: [w505] -> w489
          tunnel: [w503] -> w493 mode=indexing
          tunnel: [w502] -> w490
          tunnel: "ResetFrontImage" -> [w501]
          n140 = property class="XYGraph (strict)"(reference=w507, "PlotImages.Front"=w508) -> (reference out=w509:refnum<vi>, error out=w506:errorcluster)  [unwired: 1 in]
          n141 = call "SetCursorNamePosition XYGraph.vi"("Graph"=w509) -> ("Graph Out"=w511:refnum<vi>)
          n142 = call "SetCursorMode XYGraph.vi"("Visible"=w501, "Graph Refnum"=w511) -> ("Graph Refnum 2"=w510:refnum<vi>)  [unwired: 9 in]
          n143 = call "SetCursorNamePosition XYGraph.vi"("Graph"=w510) -> ("Graph Out"=w504:refnum<vi>)
          n144 = case shown="False" w501 {
            selector: w501 -> [w512 w518]
            tunnel: w506 -> [w516 w520]
            tunnel: [w515 w520] -> w505
            tunnel: w504 -> [w514 w519]
            tunnel: [w513 w519] -> w503
            tunnel: [w512 w518] -> w502
            frame False {
              n145 = property class="XYGraph"(reference=w514, error in=w516, "ActPaletteTool"=0 ("Palette:Active Tool")) -> (reference out=w513:refnum<vi>, error out=w515:errorcluster)
            }
            frame True {
            }
          }
        }
        n146 = Index Array(array=w493) -> (element #1=w492:refnum<vi>, element #2=w491:refnum<vi>)  [unwired: 2 in]
        n147 = call "LoadPressureAndTangents XYGraph.vi"("error in (no error)"=w489, "Red Graph"=w491, "ResetFrontImage"=w490, "Blue Graph"=w492) -> ("error out"=w488:errorcluster, "output cluster"=w479:cluster{dbl, dbl, dbl, dbl})  [unwired: 2 in]
        n148 = control-ref of="Blue Pressure"() -> (w497:refnum<vi>)
        n149 = control-ref of="Red Pressure"() -> (w496:refnum<vi>)
        n150 = Unbundle(w479) -> (w478:dbl, w477:dbl, w475:dbl, w476:dbl)
        n151 = property on="Red index" class="DigNum (strict)"("Value"=w476) -> ()  [unwired: 2 in, 2 out]
        n152 = property class="DigNum (strict)"(reference=w497, "Value"=w478) -> ()  [unwired: 1 in, 2 out]
        n153 = property class="DigNum (strict)"(reference=w496, error in=w488, "Value"=w477) -> (error out=w487:errorcluster)  [unwired: 1 out]
        n154 = property on="Blue index" class="DigNum (strict)"("Value"=w475) -> ()  [unwired: 2 in, 2 out]
        n155 = control-ref of="This VI"() -> (w485:refnum<vi>)
        n156 = property class="VI"(reference=w485, error in=w487) -> (reference out=w486:refnum<vi>, error out=w481:errorcluster, "Panel"=w484:refnum<vi>)
        n157 = property class="Pnl"(reference=w484, error in=w481, "DeferPanUpdts"=FALSE ("Defer Panel Updates")) -> (error out=w482:errorcluster)  [unwired: 1 out]
        n158 = Close Reference(reference=w486, error in (no error)=w482) -> ()  [unwired: 1 out]
      }
      event User Event {
        n159 = event-data() -> ("Tangentmode"=w525:bool, "Msg"=w524:string)  [unwired: 1 in]
        n160 = case shown="\"Set Tangent Mode\"" w524 {
          tunnel: w527 -> [_ w530]
          tunnel: w526 -> [_ w529]
          tunnel: w525 -> [_ w528]
          frame "", Default {
          }
          frame "Set Tangent Mode" {
            n161 = Build Array(w530, w529) -> (w531:refnum<vi>[])
            n162 = for {
              tunnel: picture data[5B] ("Plot Images:Front") -> [w537]
              tunnel: w531 -> [w536] mode=indexing
              tunnel: w528 -> [w533]
              n163 = property class="XYGraph (strict)"(reference=w536, "PlotImages.Front"=w537) -> (reference out=w538:refnum<vi>, error out=w535:errorcluster)  [unwired: 1 in]
              n164 = call "SetCursorNamePosition XYGraph.vi"("Graph"=w538) -> ("Graph Out"=w540:refnum<vi>)
              n165 = call "SetCursorMode XYGraph.vi"("Visible"=w533, "Graph Refnum"=w540) -> ("Graph Refnum 2"=w539:refnum<vi>)  [unwired: 9 in]
              n166 = call "SetCursorNamePosition XYGraph.vi"("Graph"=w539) -> ("Graph Out"=w534:refnum<vi>)
              n167 = case shown="False" w533 {
                selector: w533 -> [w541 w547]
                tunnel: w535 -> [w545 w549]
                tunnel: [w544 w549] -> _
                tunnel: w534 -> [w543 w548]
                tunnel: [w542 w548] -> _
                tunnel: [w541 w547] -> _
                frame False {
                  n168 = property class="XYGraph"(reference=w543, error in=w545, "ActPaletteTool"=0 ("Palette:Active Tool")) -> (reference out=w542:refnum<vi>, error out=w544:errorcluster)
                }
                frame True {
                }
              }
            }
          }
        }
      }
      event "GraphSelection(Red:F)": Value Change {
        n169 = event-data() -> ()  [unwired: 1 in, 5 out]
      }
      event "System Stop Button": Value Change {
        n170 = event-data() -> ()  [unwired: 1 in, 5 out]
      }
      event "ZoomRedBtn", "ResetRedBtn": Value Change {
        n171 = event-data() -> ()  [unwired: 1 in, 5 out]
        n172 = case shown="True" "ResetRedBtn" {
          tunnel: w557 -> [_ w566]
          tunnel: w558 -> [_ w565]
          frame False {
          }
          frame True {
            n173 = property class="XYGraph (strict)"(reference=w566, "ActPaletteTool"=5 ("Palette:Active Tool")) -> (reference out=w567:refnum<vi>)  [unwired: 1 in, 1 out]
            n174 = property class="XYGraph (strict)"(reference=w567, "ActPaletteTool"=0 ("Palette:Active Tool")) -> ()  [unwired: 1 in, 2 out]
            n175 = Enqueue Element(queue=w565, element=cluster{"Msg":string, "Data":variant} {"Msg"="Update", "Data"=variant}) -> ()  [unwired: 2 in, 3 out]
          }
        }
        n176 = case shown="True" "ZoomRedBtn" {
          tunnel: w557 -> [_ w570]
          frame False {
          }
          frame True {
            n177 = property class="XYGraph (strict)"(reference=w570, "ActPaletteTool"=2 ("Palette:Active Tool")) -> ()  [unwired: 1 in, 2 out]
            n178 = call "AE User Events.vi"("Action"=Enum_User_Events."User Event", "User Event"="TangentMode") -> ()  [unwired: 8 in, 2 out]
          }
        }
      }
      event "ZoomBlueBtn", "ResetBlueBtn": Value Change {
        n179 = event-data() -> ()  [unwired: 1 in, 5 out]
        n180 = case shown="True" "ResetBlueBtn" {
          tunnel: w574 -> [_ w589]
          tunnel: w575 -> [_ w586]
          frame False {
          }
          frame True {
            n181 = property class="XYGraph (strict)"(reference=w589, "ActPaletteTool"=5 ("Palette:Active Tool")) -> (reference out=w587:refnum<vi>)  [unwired: 1 in, 1 out]
            n182 = property class="XYGraph (strict)"(reference=w587, "ActPaletteTool"=0 ("Palette:Active Tool")) -> ()  [unwired: 1 in, 2 out]
            n183 = Enqueue Element(queue=w586, element=cluster{"Msg":string, "Data":variant} {"Msg"="Update", "Data"=variant}) -> ()  [unwired: 2 in, 3 out]
          }
        }
        n184 = case shown="True" "ZoomBlueBtn" {
          tunnel: w574 -> [_ w583]
          frame False {
          }
          frame True {
            n185 = property class="XYGraph (strict)"(reference=w583, "ActPaletteTool"=2 ("Palette:Active Tool")) -> ()  [unwired: 1 in, 2 out]
            n186 = call "AE User Events.vi"("Action"=Enum_User_Events."User Event", "User Event"="TangentMode") -> ()  [unwired: 8 in, 2 out]
          }
        }
      }
      event "Blue": Shortcut Menu Selection (User) {
        n187 = event-data() -> ("CtlRef"=w591:refnum<vi>, "ItemTag"=w594:string)  [unwired: 1 in, 5 out]
        n188 = control-ref of="Red Pressure"() -> (w593:refnum<vi>)
        n189 = control-ref of="Blue Pressure"() -> (w592:refnum<vi>)
        n190 = case shown="\"PrintImages\"" w594 {
          tunnel: w591 -> [_ w598 _ _]
          tunnel: w593 -> [_ _ w600 w608]
          tunnel: w592 -> [_ _ w601 w607]
          frame "False", Default {
          }
          frame "ZoomOut" {
            n191 = property class="XYGraph (strict)"(reference=w598, "ActPaletteTool"=5 ("Palette:Active Tool")) -> ()  [unwired: 1 in, 2 out]
          }
          frame "SaveImagePDF" {
            n192 = property class="DigNum (strict)"(reference=w600) -> ("Value"=w602:dbl)  [unwired: 1 in, 2 out]
            n193 = property class="DigNum (strict)"(reference=w601) -> ("Value"=w603:dbl)  [unwired: 1 in, 2 out]
            n194 = control-ref of="Blue"() -> (w605:refnum<vi>)
            n195 = control-ref of="Red"() -> (w604:refnum<vi>)
            n196 = call-by-ref "?"("RedPressure"=w602, "BluePressure"=w603, "Print"=FALSE, "Blue Graph Refnum"=w605, "Red Graph Refnum"=w604) -> ()  [unwired: 7 in, 2 out]
          }
          frame "PrintImages" {
            n197 = property class="DigNum (strict)"(reference=w608) -> ("Value"=w610:dbl)  [unwired: 1 in, 2 out]
            n198 = property class="DigNum (strict)"(reference=w607) -> ("Value"=w609:dbl)  [unwired: 1 in, 2 out]
            n199 = control-ref of="Blue"() -> (w612:refnum<vi>)
            n200 = control-ref of="Red"() -> (w611:refnum<vi>)
            n201 = call-by-ref "?"("RedPressure"=w610, "BluePressure"=w609, "Print"=TRUE, "Blue Graph Refnum"=w612, "Red Graph Refnum"=w611) -> ()  [unwired: 7 in, 2 out]
          }
        }
      }
      event "Red": Shortcut Menu Selection (User) {
        n202 = event-data() -> ("CtlRef"=w614:refnum<vi>, "ItemTag"=w617:string)  [unwired: 1 in, 5 out]
        n203 = control-ref of="Blue Pressure"() -> (w615:refnum<vi>)
        n204 = control-ref of="Red Pressure"() -> (w616:refnum<vi>)
        n205 = case shown="\"SaveImagePDF\"" w617 {
          tunnel: w614 -> [_ w621 _ _]
          tunnel: w616 -> [_ _ w624 w630]
          tunnel: w615 -> [_ _ w623 w631]
          frame "False", Default {
          }
          frame "ZoomOut" {
            n206 = property class="XYGraph (strict)"(reference=w621, "ActPaletteTool"=5 ("Palette:Active Tool")) -> ()  [unwired: 1 in, 2 out]
          }
          frame "SaveImagePDF" {
            n207 = property class="DigNum (strict)"(reference=w624) -> ("Value"=w625:dbl)  [unwired: 1 in, 2 out]
            n208 = property class="DigNum (strict)"(reference=w623) -> ("Value"=w626:dbl)  [unwired: 1 in, 2 out]
            n209 = control-ref of="Blue"() -> (w628:refnum<vi>)
            n210 = control-ref of="Red"() -> (w627:refnum<vi>)
            n211 = call-by-ref "?"("RedPressure"=w625, "BluePressure"=w626, "Print"=FALSE, "Blue Graph Refnum"=w628, "Red Graph Refnum"=w627) -> ()  [unwired: 7 in, 2 out]
          }
          frame "PrintImages" {
            n212 = property class="DigNum (strict)"(reference=w630) -> ("Value"=w633:dbl)  [unwired: 1 in, 2 out]
            n213 = property class="DigNum (strict)"(reference=w631) -> ("Value"=w632:dbl)  [unwired: 1 in, 2 out]
            n214 = control-ref of="Blue"() -> (w635:refnum<vi>)
            n215 = control-ref of="Red"() -> (w634:refnum<vi>)
            n216 = call-by-ref "?"("RedPressure"=w633, "BluePressure"=w632, "Print"=TRUE, "Blue Graph Refnum"=w635, "Red Graph Refnum"=w634) -> ()  [unwired: 7 in, 2 out]
          }
        }
      }
      event "Red", "Blue": Shortcut Menu Activation? {
        n217 = event-data() -> ("MenuRef"=w646:refnum<k9>)  [unwired: 1 in]
        n218 = call "AE Variables.vi"("Action"=Enum_Variables."Get Language") -> ("RingOut"=w640:u16)  [unwired: 11 in, 7 out]
        n219 = Delete Menu Items(9:w646) -> (0:w644:errorcluster, 3:w645:refnum<k9>)  [unwired: 3 in]
        n220 = case shown="0, Default" w640 {
          tunnel: [string[] ["Zoom Ud", "Gem Grafer i PDF", "Print Grafer"] ("item names") string[] ["Zoom Out", "Save Graphs as PDF", "Print Graphs"] ("item names") string[] ["Zoom Out", "Save Graphs as PDF", "Print Graphs"] ("item names")] -> w643
          frame 0, Default {
          }
          frame 1 {
          }
          frame 2 {
          }
        }
        n221 = Insert Menu Items(6:w644, 7:string[] ["ZoomOut", "SaveImagePDF", "PrintImages"] ("item tags"), 8:w643, 9:w645) -> ()  [unwired: 2 in, 3 out]
        n222 = event-data() -> ()  [unwired: 2 in, 1 out]
      }
      event Pane Size {
        n223 = event-data() -> ()  [unwired: 1 in, 1 out]
        n224 = Enqueue Element(queue=w654, element=cluster{"Msg":string, "Data":variant} {"Msg"="Update", "Data"=variant}) -> ()  [unwired: 2 in, 3 out]
      }
    }
  }
  n225 = call <vilib>:"General Error Handler.vi"("error in (no error)"=w9) -> ()  [unwired: 10 in, 5 out]
  n226 = Destroy User Event(user event=w8, error in=w9) -> (error out=w10:errorcluster)
  n227 = Unregister For Events(event registration refnum=w11, error in=w10) -> (error out=w7:errorcluster)
  n228 = Release Queue(queue="Queue", force destroy? (F)=TRUE, error in (no error)=w14) -> ()  [unwired: 3 out]
  n229 = call <vilib>:"Clear Errors.vi"("error in (no error)"=w7) -> ()  [unwired: 6 in, 1 out]
  "Red" <- w1
  "Blue" <- w1
